vi "Exemple_Metrics_Mutual_Info_Score.vi"() -> ()   [LabVIEW 2020]
uses:
  Objet/3 - Model selection and evaluation/3.3 - Metrics and scoring/mutual_info_score/Mutual_Info_Score.vi
panel:
  out "Score":string
  out "error out":errorcluster caption="sortie d'erreur"
  in  "mutual_info_score":T1
  in  "labels_pred":string[][](array[string])=[["0"], ["0"], ["1"], ["1"]]
  in  "labels_true":string[][](array[string])=[["0"], ["0"], ["1"], ["1"]]
  in  "error in (no error)":errorcluster caption="entrée d'erreur (pas d'erreur)"
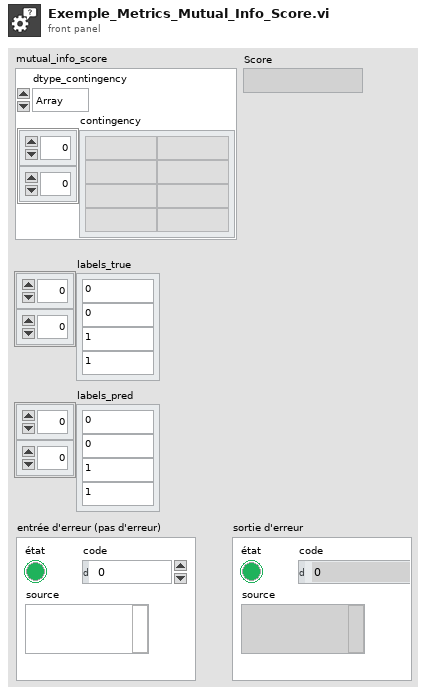
[diagram p1: front panel]
types:
  T1 = cluster{"dtype_contingency":enum16{"Array", "Sparse"}, "contingency":string[][]}
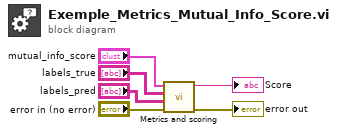
[diagram p0: block diagram]
diagram:
  n1 = call-poly "Metrics and scoring.vi"("error in (no error)"="error in (no error)", "labels_pred"="labels_pred", "labels_true"="labels_true", "mutual_info_score"="mutual_info_score") -> ("error out"=→"error out":errorcluster, "Score"=→"Score":string)  [unwired: 6 in]
